vi "Check Data Model.vi"(8 "error in":errorcluster, 11 "Super Data Model in":refnum<class "Super Data Model.lvclass">) -> (0 "error out":errorcluster, 3 "Super Data Model out":refnum<class "Super Data Model.lvclass">)   [LabVIEW 2013, in "Modbus Library - Advance.lvlib" / "Super Data Model.lvclass"]
uses:
  Super Data Model.lvclass
  Standard Data Model/Standard Data Model.lvclass
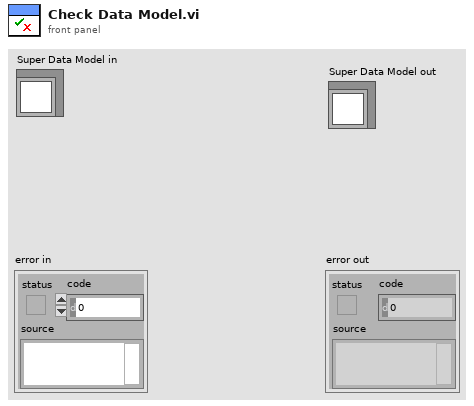
[diagram p1: front panel]
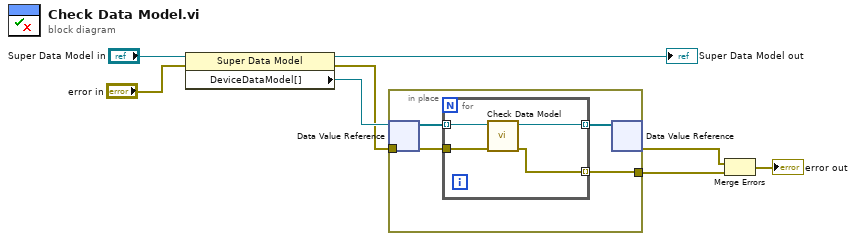
[diagram p0: block diagram]
diagram:
  n1 = property class="Super Data Model"(reference="Super Data Model in", error in="error in") -> (reference out=→"Super Data Model out":refnum<class "Super Data Model.lvclass">, error out=w4:errorcluster, "DeviceDataModel[]"=w6:refnum<data-value>)
  n2 = in-place {
    in-place-border: w4 -> [w10]
    in-place-border: [w9] -> w2
    n3 = in-place-dvr #1(w6) -> (w12:refnum<class "Standard Data Model.lvclass">[])  [unwired: 1 out]
    n4 = for {
      tunnel: w12 -> [w16] mode=indexing
      tunnel: [w15] -> w11 mode=indexing
      tunnel: w10 -> [w14]
      tunnel: [w13] -> w9 mode=indexing
      n5 = call-dynamic "Check Data Model.vi"("error in"=w14, "device data model in"=w16) -> ("error out"=w13:errorcluster, "device data model out"=w15:refnum<class "Standard Data Model.lvclass">)  [unwired: 8 in]
    }
    n6 = in-place-dvr #1(w11) -> (w3:errorcluster)  [unwired: 1 out]
  }
  n7 = Merge Errors(w3, w2) -> (→"error out":errorcluster)
